vi "Continous Wave DAC Dual Output.vi"() -> ()   [LabVIEW 2012]
doc: "This example demonstrates how to continuously re-generate analog output data from a buffer in your computer's memory.\n\nRefer to your device documentation for pinouts and hardware capabilities."
uses:
  <vilib>/DAQmx/write.llb/DAQmx Write (Analog 1D Wfm NChan NSamp).vi
  <vilib>/DAQmx/create/channels.llb/DAQmx Create Channel (AO-Voltage-Basic).vi
  <vilib>/DAQmx/configure/timing.llb/DAQmx Timing (Sample Clock).vi
  <vilib>/DAQmx/miscellaneous.llb/DAQmx Fill In Error Info.vi
  <resource>/objmgr/daqmx.rc
  <vilib>/measure/NI_MABase.lvlib
panel:
  out "Waveform Graph 2":waveform(dbl)[](graph)=[{"t0"=timestamp(0 s since 1904-01-01), "dt"=0.001, "Y"=[]}]
  in  "Output Array 2":T1(array[cluster])=[{"Waveform Type"=0, "Amplitude"=1.0, "Frequency"=10.0, "Phase"=0.0}] {"Frequency" format="%0.2p"; "Amplitude" format="%0.2p"; "Waveform Type" items=["Sine Wave", "Triangle Wave", "Square Wave", "Sawtooth Wave"]}
  in  "Sample Rate 2":dbl=1000.0
  in  "Sample Clock Source 2":tag="OnboardClock"
  in  "Max Voltage 2":dbl=5.0
  in  "Min Voltage 2":dbl=-5.0
  in  "Physical Channel(s) 2":tag="Dev1/ao0"
  out "Actual Sample Rate 2":dbl=1000.0 format="%0.2f"
  in  "Output Array":T2(array[cluster])=[{"Waveform Type"=0, "Amplitude"=1.0, "Frequency"=10.0}] {"Frequency" format="%0.2p"; "Amplitude" format="%0.2p"; "Waveform Type" items=["Sine Wave", "Triangle Wave", "Square Wave", "Sawtooth Wave"]}
  in  "Number of Samples":i32=1000
  in  "Stop":bool
  out "Waveform Graph":waveform(dbl)[](graph)=[{"t0"=timestamp(0 s since 1904-01-01), "dt"=0.001, "Y"=[]}]
  in  "Sample Rate":dbl=1000.0
  in  "Sample Clock Source":tag="OnboardClock"
  in  "Max Voltage":dbl=5.0
  in  "Min Voltage":dbl=-5.0
  in  "Physical Channel(s)":tag="Dev1/ao0"
  out "Actual Sample Rate":dbl=1000.0 format="%0.2f"
  # "Channel Settings"
  # "Output"
  # "Timing and Buffer Settings"
  # "Waveform Settings"
  # "The number of elements in the waveform array\nmust equal the number of channels in the task."
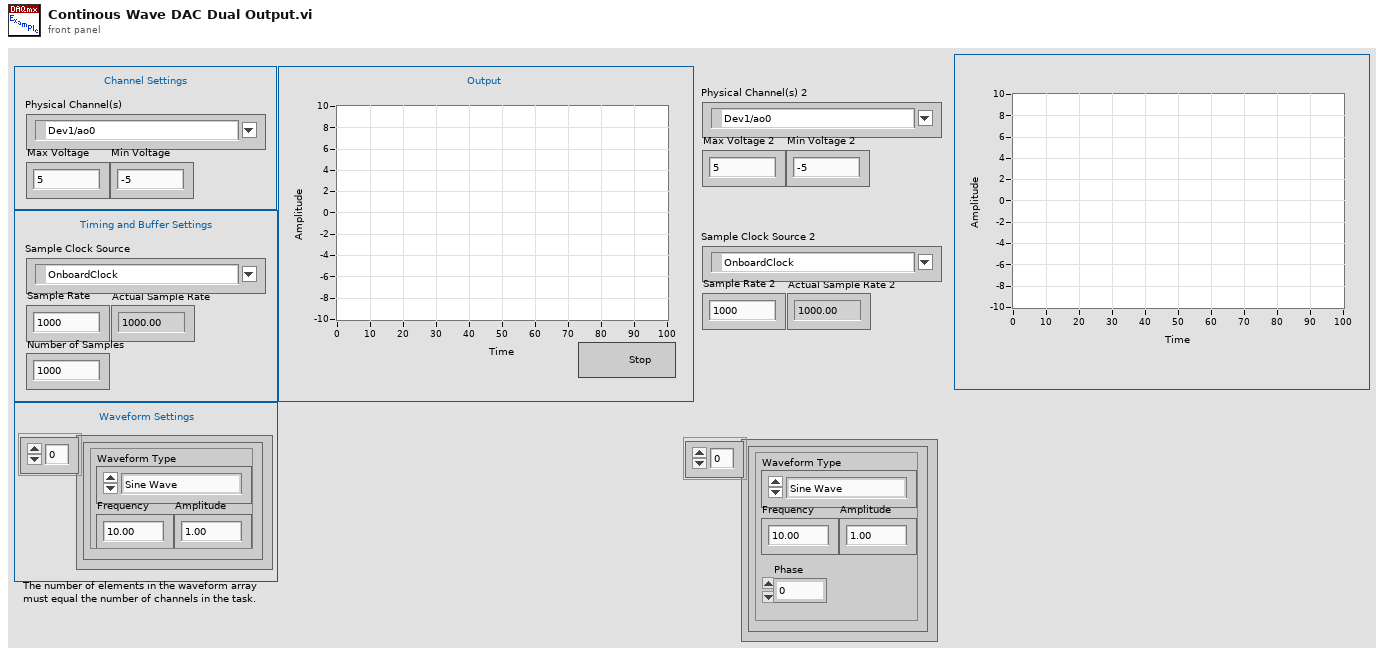
[diagram p1: front panel]
types:
  T1 = cluster{"Waveform Type":u16, "Amplitude":dbl, "Frequency":dbl, "Phase":dbl}[]
  T2 = cluster{"Waveform Type":u16, "Amplitude":dbl, "Frequency":dbl}[]
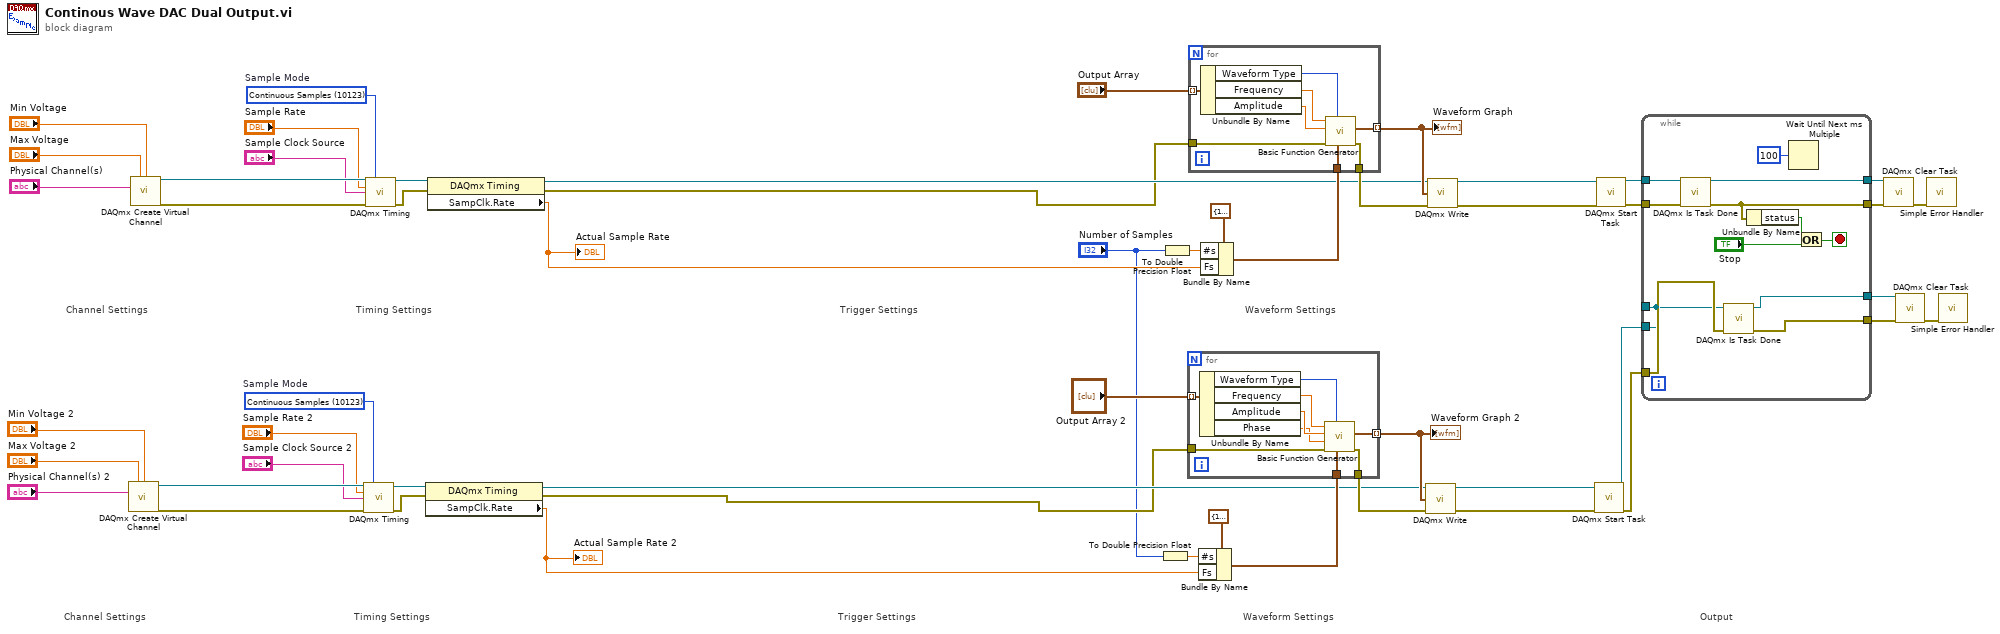
[diagram p0: block diagram]
diagram:
  w29 = 10123 items=["Finite Samples"=10178, "Continuous Samples"=10123, "Hardware Timed Single Point"=12522]  # Sample Mode
  w51 = 10123 items=["Finite Samples"=10178, "Continuous Samples"=10123, "Hardware Timed Single Point"=12522]  # Sample Mode
  # "Output"
  # "Trigger Settings"
  # "Waveform Settings"
  # "Timing Settings"
  # "Channel Settings"
  # "Trigger Settings"
  # "Waveform Settings"
  # "Timing Settings"
  # "Channel Settings"
  n1 = call-poly <vilib>:"DAQmx Create Virtual Channel.vi"("maximum value"="Max Voltage 2", "minimum value"="Min Voltage 2", "physical channels"="Physical Channel(s) 2") -> ("task out"=w27:refnum<k21>, "error out"=w28:errorcluster)  [unwired: 11 in]
  n2 = call-poly <vilib>:"DAQmx Create Virtual Channel.vi"("maximum value"="Max Voltage", "minimum value"="Min Voltage", "physical channels"="Physical Channel(s)") -> ("task out"=w49:refnum<k21>, "error out"=w50:errorcluster)  [unwired: 11 in]
  n3 = call-poly <vilib>:"DAQmx Timing.vi"("task/channels in"=w27, "sample mode"=w29, "rate"="Sample Rate 2", "source"="Sample Clock Source 2", "error in"=w28) -> ("task out"=w31:refnum<k21>, "error out"=w30:errorcluster)  [unwired: 9 in]
  n4 = call-poly <vilib>:"DAQmx Timing.vi"("task/channels in"=w49, "sample mode"=w51, "rate"="Sample Rate", "source"="Sample Clock Source", "error in"=w50) -> ("task out"=w53:refnum<k21>, "error out"=w52:errorcluster)  [unwired: 9 in]
  n5 = property class="DAQmx Timing"(reference=w31, error in=w30) -> (reference out=w9:refnum<k21>, error out=w8:errorcluster, "SampClk.Rate"=w19:dbl)
  "Actual Sample Rate 2" <- w19
  n6 = property class="DAQmx Timing"(reference=w53, error in=w52) -> (reference out=w11:refnum<k21>, error out=w10:errorcluster, "SampClk.Rate"=w39:dbl)
  "Actual Sample Rate" <- w39
  n7 = To Double Precision Float(number="Number of Samples") -> (double precision float=w12:dbl)
  n8 = To Double Precision Float(number="Number of Samples") -> (double precision float=w32:dbl)
  n9 = Bundle By Name(cluster=cluster{"Fs":dbl, "#s":dbl} {"Fs"=1000.0, "#s"=1000.0} ("sampling info"), "#s"=w12, "Fs"=w19) -> (w18:cluster{"Fs":dbl, "#s":dbl})
  n10 = for {
    tunnel: w8 -> [w62]
    tunnel: w18 -> [w61]
    tunnel: [w60] -> w15
    tunnel: "Output Array 2" -> [w59] mode=indexing
    tunnel: [w55] -> w13 mode=indexing
    n11 = Unbundle By Name(w59) -> ("Waveform Type"=w58:u16, "Frequency"=w57:dbl, "Amplitude"=w56:dbl, "Phase"=w54:dbl)
    n12 = call <vilib>:"Basic Function Generator.vi"("sampling info"=w61, "signal type"=w58, "error in (no error)"=w62, "phase"=w54, "amplitude"=w56, "frequency"=w57) -> ("error out"=w60:errorcluster, "signal out"=w55:waveform(dbl))  [unwired: 3 in, 1 out]
  }
  "Waveform Graph 2" <- w13
  n13 = Bundle By Name(cluster=cluster{"Fs":dbl, "#s":dbl} {"Fs"=1000.0, "#s"=1000.0} ("sampling info"), "#s"=w32, "Fs"=w39) -> (w38:cluster{"Fs":dbl, "#s":dbl})
  n14 = for {
    tunnel: w10 -> [w70]
    tunnel: w38 -> [w69]
    tunnel: [w68] -> w35
    tunnel: "Output Array" -> [w67] mode=indexing
    tunnel: [w63] -> w33 mode=indexing
    n15 = Unbundle By Name(w67) -> ("Waveform Type"=w66:u16, "Frequency"=w65:dbl, "Amplitude"=w64:dbl)
    n16 = call <vilib>:"Basic Function Generator.vi"("sampling info"=w69, "signal type"=w66, "error in (no error)"=w70, "amplitude"=w64, "frequency"=w65) -> ("error out"=w68:errorcluster, "signal out"=w63:waveform(dbl))  [unwired: 4 in, 1 out]
  }
  "Waveform Graph" <- w33
  n17 = call-poly <vilib>:"DAQmx Write.vi"("task/channels in"=w9, "data"=w13, "error in"=w15) -> ("task out"=w17:refnum<k21>, "error out"=w16:errorcluster)  [unwired: 10 in, 1 out]
  n18 = call-poly <vilib>:"DAQmx Write.vi"("task/channels in"=w11, "data"=w33, "error in"=w35) -> ("task out"=w37:refnum<k21>, "error out"=w36:errorcluster)  [unwired: 10 in, 1 out]
  n19 = call <vilib>:"DAQmx Start Task.vi"("task/channels in"=w17, "error in"=w16) -> ("task out"=w1:refnum<k21>, "error out"=w2:errorcluster)  [unwired: 12 in]
  n20 = call <vilib>:"DAQmx Start Task.vi"("task/channels in"=w37, "error in"=w36) -> ("task out"=w6:refnum<k21>, "error out"=w5:errorcluster)  [unwired: 12 in]
  n21 = while {
    tunnel: w6 -> [w82]
    tunnel: w5 -> [w81]
    tunnel: [w78] -> w47
    tunnel: [w79] -> w48
    tunnel: [w71] -> _
    tunnel: [w74] -> w4
    tunnel: [w73] -> w3
    tunnel: w2 -> [w72]
    tunnel: w1 -> [w71]
    stop <- w80 stop-if-true
    n22 = call <vilib>:"DAQmx Is Task Done.vi"("task/channels in"=w82, "error in"=w81) -> ("task out"=w79:refnum<k21>, "error out"=w78:errorcluster)  [unwired: 11 in, 1 out]
    n23 = call <vilib>:"DAQmx Is Task Done.vi"("task/channels in"=w71, "error in"=w72) -> ("task out"=w74:refnum<k21>, "error out"=w73:errorcluster)  [unwired: 11 in, 1 out]
    n24 = Unbundle By Name(w78) -> ("status"=w77:bool)
    n25 = Wait Until Next ms Multiple(millisecond multiple=u32 100) -> ()  [unwired: 1 out]
    n26 = Or(x=w77, y="Stop") -> (x .or. y?=w80:bool)
  }
  n27 = call <vilib>:"DAQmx Clear Task.vi"("task in"=w48, "error in"=w47) -> ("error out"=w46:errorcluster)  [unwired: 13 in]
  n28 = call <vilib>:"DAQmx Clear Task.vi"("task in"=w4, "error in"=w3) -> ("error out"=w26:errorcluster)  [unwired: 13 in]
  n29 = call <vilib>:"Simple Error Handler.vi"("error in (no error)"=w46) -> ()  [unwired: 4 in, 5 out]
  n30 = call <vilib>:"Simple Error Handler.vi"("error in (no error)"=w26) -> ()  [unwired: 4 in, 5 out]
